vi "Measure-SM1000-modulation.vi"(8 "error in (no error)":errorcluster, 9 "Device index":i32, 10 "File path":path, 11 "SM1000-control in":T1) -> (0 "error out":errorcluster, 2 "Modulation data":i32[][](array[numeric]), 3 "SM1000-control out":T1)   [LabVIEW 2013, in "MaterialCharacterization.lvlib" / "MC-SM1000.lvclass"]
uses:
  MC-SM1000.lvclass
  Object-reference.ctl
  <vilib>/DAQmx/read.llb/DAQmx Read (Digital 1D U32 1Chan NSamp).vi
  <vilib>/DAQmx/miscellaneous.llb/DAQmx Fill In Error Info.vi
panel:
  out "Graph":i32[][](graph)
  in  "Start job":bool
  out "Job busy":bool
  in  "Stop":bool
  out "Elapsed time":dbl caption="Elapsed time [ms]" format="%.2f"
  out "Initialized":bool
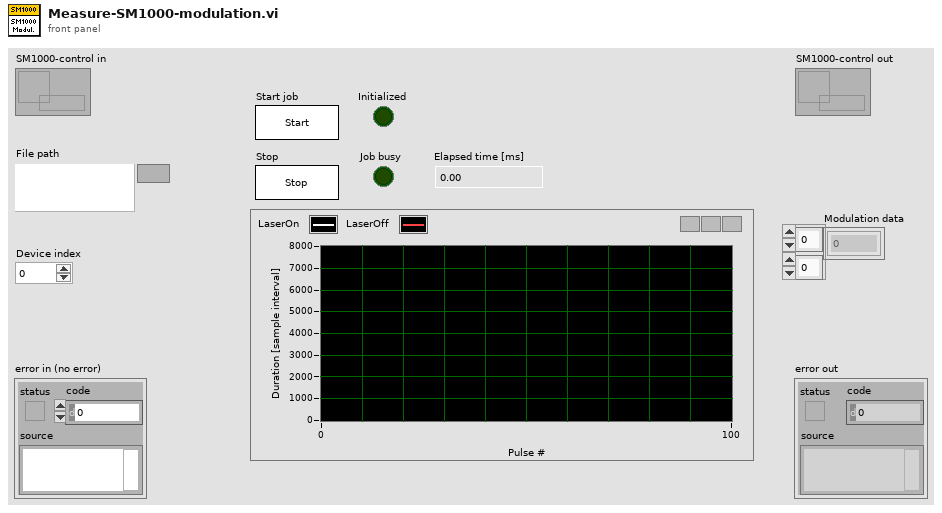
[diagram p1: front panel]
types:
  T1 = typedef "MaterialCharacterization.lvlib/MC-SM1000.lvclass/Object-reference.ctl" = refnum<data-value>
  T2 = enum8{"Enabled", "Disabled", "Disabled and Grayed Out"}
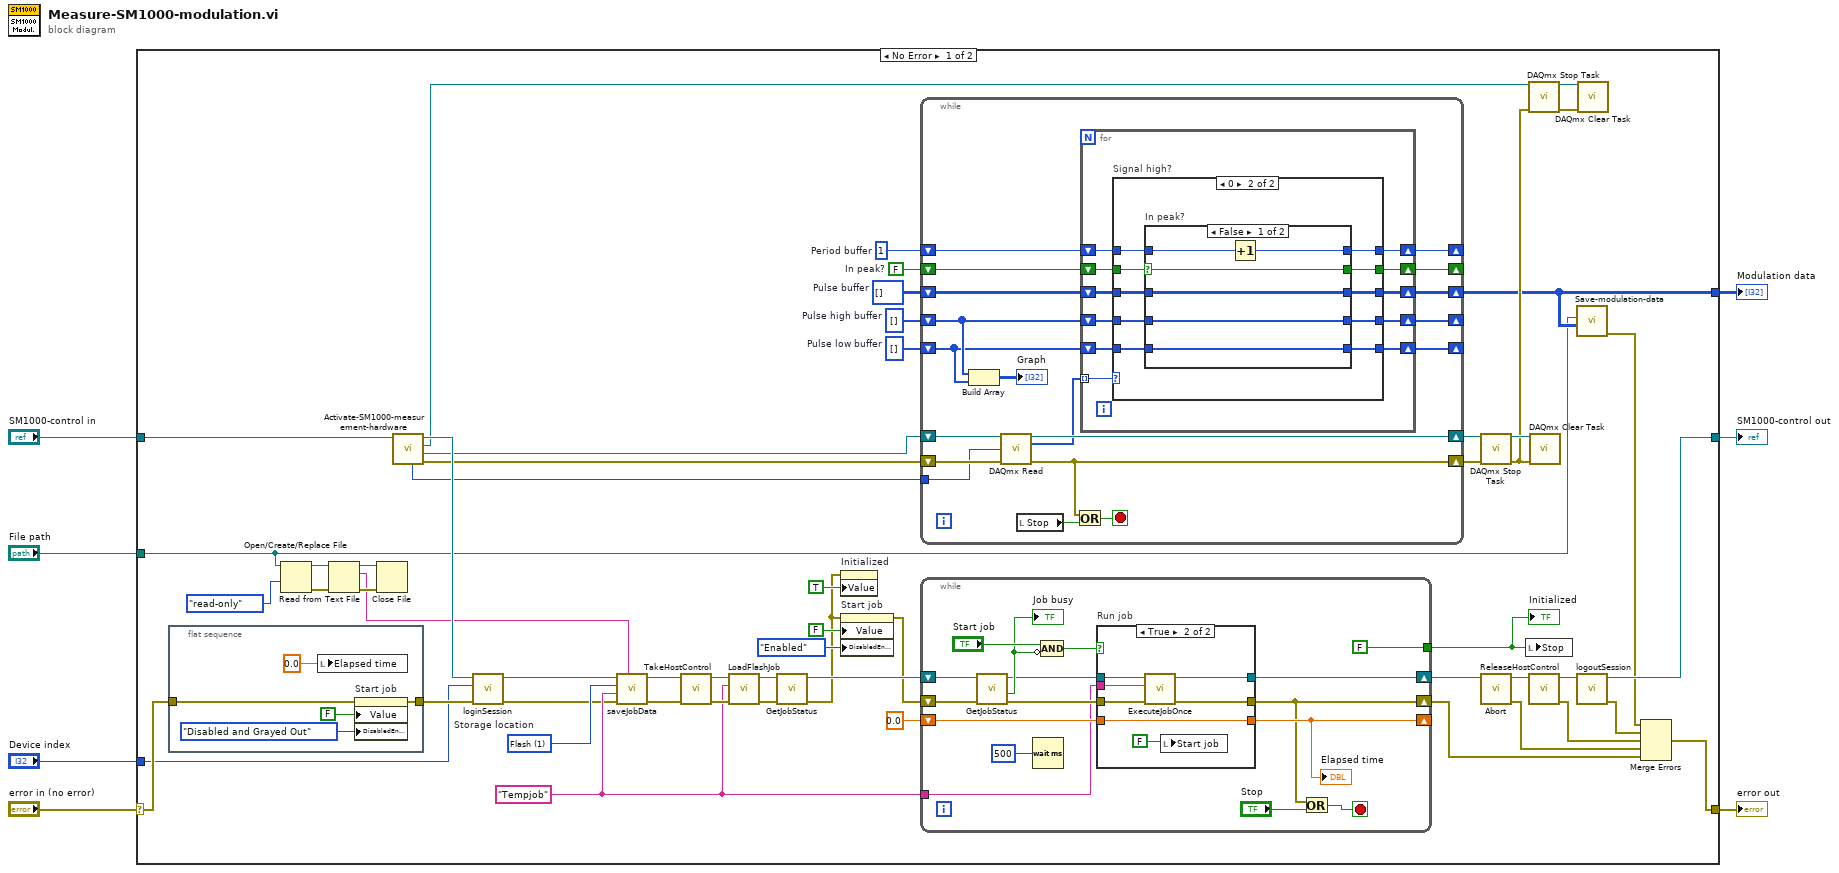
[diagram p0: block diagram]
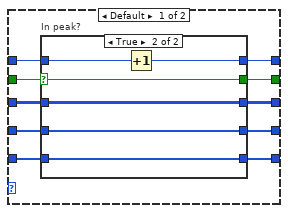
[diagram p2: hidden frame]
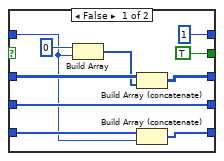
[diagram p3: hidden frame]
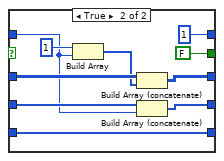
[diagram p4: hidden frame]
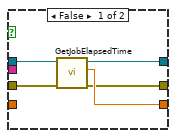
[diagram p5: hidden frame]
diagram:
  n1 = case shown="No Error" "error in (no error)" {
    selector: "error in (no error)" -> [w41 w180]
    tunnel: [w52 w180] -> w6
    tunnel: [w50 w179] -> w4
    tunnel: "SM1000-control in" -> [w37 w179]
    tunnel: "File path" -> [w10 _]
    tunnel: "Device index" -> [w40 _]
    tunnel: [w17 _] -> w1
    frame No Error {
      w19 = i32[] []  # Pulse low buffer
      w20 = i32[] []  # Pulse high buffer
      w21 = i32[][] []  # Pulse buffer
      w23 = 1  # Period buffer
      w22 = FALSE  # In peak?
      w59 = u16 1 items=["Flash"=1, "USB"=2]  # Storage location
      w56 = "Tempjob"
      n2 = flat-sequence {
        tunnel: [w148] -> w42
        tunnel: w41 -> [w147]
        frame #0 {
          n3 = local write "Elapsed time"(0.0 ("Elapsed time")) -> ()
          n4 = property on="Start job" class="Bool (strict)"(error in=w147, "Value"=FALSE, "DisabledEnum"=T2."Disabled and Grayed Out" ("Disabled")) -> (error out=w148:errorcluster)  [unwired: 1 in, 1 out]
        }
      }
      n5 = Open/Create/Replace File(file path (use dialog)=w10, access (0:read/write)=enum16{"read/write", "read-only", "write-only"}."read-only") -> (refnum out=w15:refnum<file>, error out=w12:errorcluster)  [unwired: 4 in, 1 out]
      n6 = Read from Text File(file (use dialog)=w15, error in=w12) -> (refnum out=w14:refnum<file>, text=w8:string, error out=w13:errorcluster)  [unwired: 2 in, 1 out]
      n7 = Close File(refnum=w14, error in=w13) -> ()  [unwired: 2 out]
      n8 = call "Activate-SM1000-measurement-hardware.vi"("SM1000-control in"=w37) -> ("error out"=w30:errorcluster, "Signal"=w32:refnum<k21>, "Timing"=w28:refnum<k21>, "SM1000-control out"=w36:T1, "Batch size"=w31:i32)  [unwired: 6 in]
      n9 = call "loginSession.vi"("error in (no error)"=w42, "Device index"=w40, "SM1000-control in"=w36) -> ("error out"=w9:errorcluster, "SM1000-control out"=w47:T1)  [unwired: 7 in]
      n10 = call "saveJobData.vi"("Job data xml"=w8, "error in (no error)"=w9, "File name wo extension"=w56, "Storage location"=w59, "SM1000-control in"=w47) -> ("error out"=w34:errorcluster, "SM1000-control out"=w35:T1)  [unwired: 5 in]
      n11 = call "TakeHostControl.vi"("error in (no error)"=w34, "SM1000-control in"=w35) -> ("error out"=w61:errorcluster, "SM1000-control out"=w60:T1)  [unwired: 8 in]
      n12 = call "LoadFlashJob.vi"("error in (no error)"=w61, "Job name wo extension"=w56, "SM1000-control in"=w60) -> ("error out"=w63:errorcluster, "SM1000-control out"=w62:T1)  [unwired: 7 in]
      n13 = call "GetJobStatus.vi"("error in (no error)"=w63, "SM1000-control in"=w62) -> ("error out"=w38:errorcluster, "SM1000-control out"=w58:T1)  [unwired: 7 in, 1 out]
      n14 = property on="Initialized" class="Bool (strict)"(error in=w38, "Value"=TRUE ("Initialized")) -> ()  [unwired: 1 in, 2 out]
      n15 = property on="Start job" class="Bool (strict)"(error in=w38, "Value"=FALSE, "DisabledEnum"=T2."Enabled" ("Disabled")) -> (error out=w46:errorcluster)  [unwired: 1 in, 1 out]
      n16 = while {
        tunnel: w31 -> [w80]
        shift-right: [w79] -> w26
        shift-left: w32 -> [w82]
        shift-right: [w76] -> w25
        shift-left: w30 -> [w81]
        shift-right: [w73] -> _
        shift-left: w23 -> [w74]
        shift-right: [w71] -> _
        shift-left: w22 -> [w72]
        shift-right: [w69] -> w17
        shift-left: w21 -> [w70]
        shift-right: [w68] -> _
        shift-left: w20 -> [w65]
        shift-right: [w67] -> _
        shift-left: w19 -> [w64]
        stop <- w78 stop-if-true
        n17 = Build Array(w65, w64) -> (→"Graph":i32[][])
        n18 = call-poly <vilib>:"DAQmx Read.vi"("task/channels in"=w82, "number of samples per channel"=w80, "error in"=w81) -> ("task out"=w79:refnum<k21>, "data"=w75:u32[], "error out"=w76:errorcluster)  [unwired: 10 in]
        n19 = local read "Stop"() -> (w77:bool)
        n20 = Or(x=w76, y=w77) -> (x .or. y?=w78:bool)
        n21 = for {
          tunnel: w75 -> [w87] mode=indexing
          shift-right: [w91] -> w69
          shift-left: w70 -> [w92]
          shift-right: [w89] -> w73
          shift-left: w74 -> [w90]
          shift-right: [w88] -> w71
          shift-left: w72 -> [w93]
          shift-right: [w84] -> w68
          shift-left: w65 -> [w86]
          shift-right: [w83] -> w67
          shift-left: w64 -> [w85]
          n22 = case "Signal high?" shown="0" w87 {
            tunnel: w93 -> [w103 w129]
            tunnel: w92 -> [w102 w128]
            tunnel: [w101 w127] -> w91
            tunnel: w90 -> [w100 w126]
            tunnel: [w99 w125] -> w89
            tunnel: [w98 w124] -> w88
            tunnel: w86 -> [w97 w123]
            tunnel: w85 -> [w96 w121]
            tunnel: [w95 w122] -> w84
            tunnel: [w94 w120] -> w83
            frame Default {
              n23 = case "In peak?" shown="True" w103 {
                selector: w103 -> [_ w117]
                tunnel: w102 -> [w111 w119]
                tunnel: [w110 w119] -> w101
                tunnel: w100 -> [w104 w118]
                tunnel: [1 w116] -> w99
                tunnel: [TRUE w117] -> w98
                tunnel: w97 -> [w107 w115]
                tunnel: w96 -> [w106 w114]
                tunnel: [w107 w115] -> w95
                tunnel: [w105 w114] -> w94
                frame False {
                  n24 = Build Array(0, w104) -> (w109:i32[])
                  n25 = Build Array (concatenate)(w111, w109) -> (w110:i32[][])
                  n26 = Build Array (concatenate)(w106, w104) -> (w105:i32[])
                }
                frame True {
                  n27 = Increment(x=w118) -> (x+1=w116:i32)
                }
              }
            }
            frame 0 {
              n28 = case "In peak?" shown="False" w129 {
                selector: w129 -> [w133 _]
                tunnel: w128 -> [w135 w143]
                tunnel: [w135 w142] -> w127
                tunnel: w126 -> [w134 w136]
                tunnel: [w132 1] -> w125
                tunnel: [w133 FALSE] -> w124
                tunnel: w123 -> [w131 w139]
                tunnel: [w131 w138] -> w122
                tunnel: w121 -> [w130 w137]
                tunnel: [w130 w137] -> w120
                frame False {
                  n29 = Increment(x=w134) -> (x+1=w132:i32)
                }
                frame True {
                  n30 = Build Array(1, w136) -> (w141:i32[])
                  n31 = Build Array (concatenate)(w143, w141) -> (w142:i32[][])
                  n32 = Build Array (concatenate)(w139, w136) -> (w138:i32[])
                }
              }
            }
          }
        }
      }
      n33 = while {
        shift-right: [w151] -> w33
        shift-left: w46 -> [w165]
        shift-right: [w152] -> w48
        shift-left: w58 -> [w166]
        shift-right: [w156] -> _
        shift-left: 0.0 ("Elapsed time") -> [w157]
        tunnel: w56 -> [w155]
        tunnel: [FALSE] -> w44
        stop <- w160 stop-if-true
        n34 = call "GetJobStatus.vi"("error in (no error)"=w165, "SM1000-control in"=w166) -> ("error out"=w159:errorcluster, "Busy?"=w162:bool, "SM1000-control out"=w158:T1)  [unwired: 7 in]
        "Job busy" <- w162
        n35 = Wait (ms)(milliseconds to wait=u32 500) -> ()  [unwired: 1 out]
        n36 = Compound Arithmetic op=AND("Start job", invert w162) -> (w163:bool)
        n37 = case "Run job" shown="True" w163 {
          tunnel: w159 -> [w169 w175]
          tunnel: [w167 w174] -> w151
          tunnel: [w168 w173] -> w152
          tunnel: w158 -> [w171 w176]
          tunnel: [w170 w178] -> w156
          tunnel: w157 -> [_ w178]
          tunnel: w155 -> [_ w177]
          frame False {
            n38 = call "GetJobElapsedTime.vi"("error in (no error)"=w169, "SM1000-control in"=w171) -> ("error out"=w167:errorcluster, "Elapsed time"=w170:dbl, "SM1000-control out"=w168:T1)  [unwired: 7 in]
          }
          frame True {
            n39 = call "ExecuteJobOnce.vi"("error in (no error)"=w175, "Job name wo extension"=w177, "SM1000-control in"=w176) -> ("error out"=w174:errorcluster, "SM1000-control out"=w173:T1)  [unwired: 7 in]
            n40 = local write "Start job"(FALSE) -> ()
          }
        }
        "Elapsed time" <- w156
        n41 = Or(x=w151, y="Stop") -> (x .or. y?=w160:bool)
      }
      "Initialized" <- w44
      n42 = call <vilib>:"DAQmx Stop Task.vi"("task/channels in"=w26, "error in"=w25) -> ("task out"=w24:refnum<k21>, "error out"=w18:errorcluster)  [unwired: 12 in]
      n43 = call "Abort.vi"("SM1000-control in"=w48) -> ("error out"=w53:errorcluster, "SM1000-control out"=w55:T1)  [unwired: 9 in]
      n44 = local write "Stop"(w44) -> ()
      n45 = call <vilib>:"DAQmx Stop Task.vi"("task/channels in"=w28, "error in"=w18) -> ("task out"=w27:refnum<k21>, "error out"=w29:errorcluster)  [unwired: 12 in]
      n46 = call "ReleaseHostControl.vi"("SM1000-control in"=w55) -> ("error out"=w54:errorcluster, "SM1000-control out"=w51:T1)  [unwired: 9 in]
      n47 = call <vilib>:"DAQmx Clear Task.vi"("task in"=w24, "error in"=w18) -> ()  [unwired: 13 in, 1 out]
      n48 = call "Save-modulation-data.vi"("Modulation data"=w17, "File path"=w10) -> ("error out"=w16:errorcluster)  [unwired: 9 in]
      n49 = call "logoutSession.vi"("SM1000-control in"=w51) -> ("error out"=w49:errorcluster, "SM1000-control out"=w50:T1)  [unwired: 9 in]
      n50 = call <vilib>:"DAQmx Clear Task.vi"("task in"=w27, "error in"=w29) -> ()  [unwired: 13 in, 1 out]
      n51 = Merge Errors(w16, w49, w54, w53, w33) -> (w52:errorcluster)
    }
    frame Error {
    }
  }
  "error out" <- w6
  "SM1000-control out" <- w4
  "Modulation data" <- w1
